vi "read_Rx_pulses_tdms_to data.vi"(8 "error in (no error)":errorcluster, 10 "num of pulses to read":i64=-1, 11 "pulse_gen_and_detect_p2p in":refnum<class "pulse_gen_and_detect_p2p.lvclass">) -> (0 "error out":errorcluster, 2 "PDWout":T1(array[cluster]), 3 "pulse_gen_and_detect_p2p out":refnum<class "pulse_gen_and_detect_p2p.lvclass">)   [LabVIEW 2021, in "pulse_gen_and_detect_p2p.lvclass"]
uses:
  pulse_gen_and_detect_p2p.lvclass
  fpga/vis/pulse detector/PDW interpoter params.ctl
  pulse_gen_and_detect_p2p.lvclass/pulse_gen_and_detect_p2p.ctl
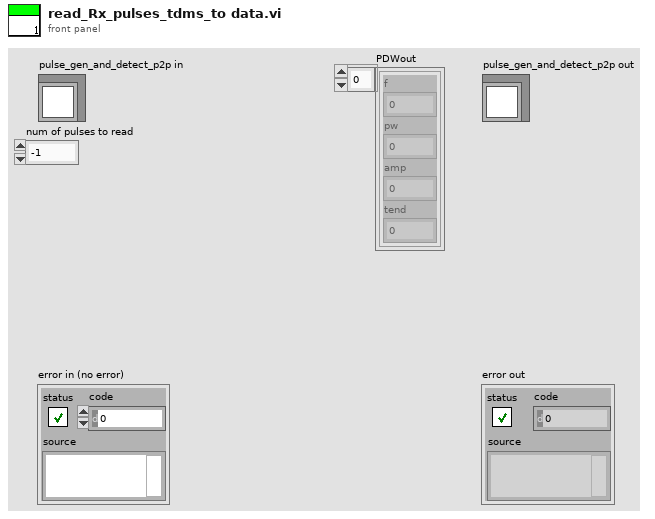
[diagram p1: front panel]
types:
  T1 = cluster{"f":dbl, "pw":dbl, "amp":dbl, "tend":dbl}[]
  T2 = typedef "PDW interpoter params.ctl" = cluster{"Fs (Hz)":dbl, "fft size ":u32, "F base (Hz)":dbl, "min AMP (dB)":dbl, "PW low bar (fft cycle)":dbl, "Pw high bar (fft cycle)":dbl, "lo likege removal (fft bin)":i32, "max gap (fft cycle)":dbl}
  T3 = enum16{"open", "open or create", "create or replace", "create", "open (read-only)"}
  T4 = cluster{"min PW (fft cycels)":u16, "max PW (fft cycels)":u16, "max gap (fft cycels)":u8, "detection bar (liniar amp)":fxp<+,64,63>, "peak detect":bool}
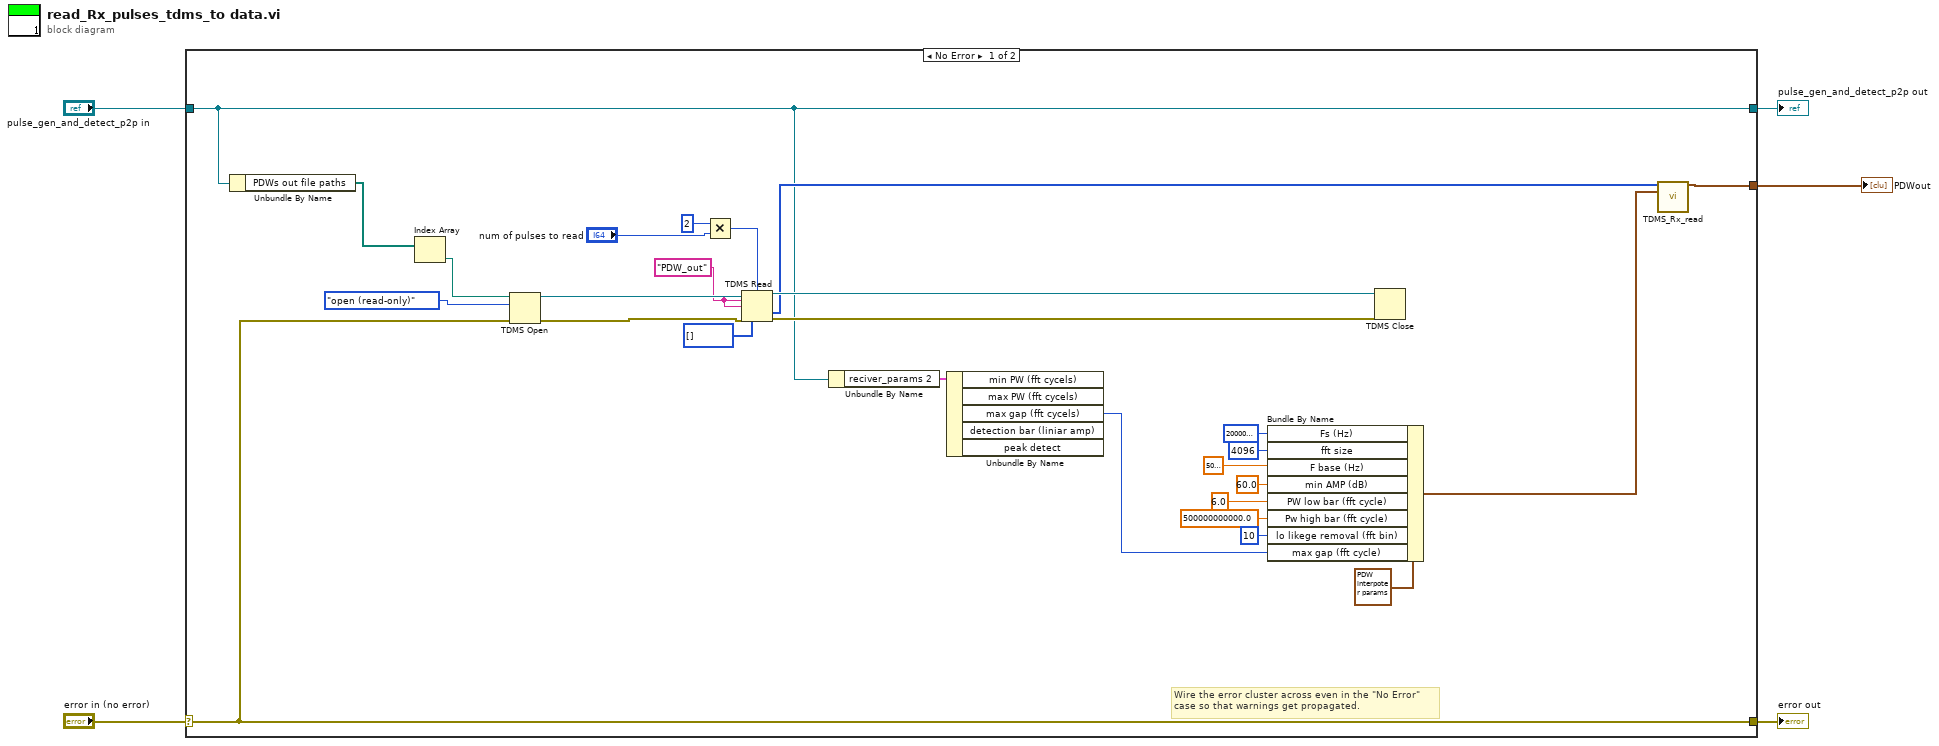
[diagram p0: block diagram]
diagram:
  n1 = case shown="No Error" "error in (no error)" {
    selector: "error in (no error)" -> [w29 w34]
    tunnel: [w29 w34] -> w4
    tunnel: [w9 w33] -> w2
    tunnel: "pulse_gen_and_detect_p2p in" -> [w9 w33]
    tunnel: [w18 _] -> w1
    frame No Error {
      w24 = "PDW_out" ("group name in")
      # "Wire the error cluster across even in the \"No Error\"\ncase so that warnings get propagated."
      n2 = Unbundle By Name(w9) -> ("PDWs out file paths"=w27:path[])
      n3 = Index Array(array=w27) -> (element=w26:path)  [unwired: 1 in]
      n4 = TDMS Open(8:w29, 10:T3."open (read-only)" ("operation (0:open)"), 11:w26) -> (0:w28:errorcluster, 3:w32:refnum<k34>)  [unwired: 4 in]
      n5 = Multiply(x=i64 2, y="num of pulses to read") -> (x*y=w20:i64)
      n6 = TDMS Read(0:w32, 2:w20, 5:w24, 7:w24, 11:w28, 12:u64[] []) -> (4:w31:refnum<k34>, 10:w19:u64[], 15:w23:errorcluster)  [unwired: 2 in, 3 out]
      n7 = Unbundle By Name(w9) -> ("reciver_params 2"=w17:T4)
      n8 = Unbundle By Name(w17) -> ("max gap (fft cycels)"=w14:u8)  [unwired: 4 out]
      n9 = Bundle By Name(cluster=T2 {"Fs (Hz)"=200000000.0, "fft size "=4096, "F base (Hz)"=2000000000.0, "min AMP (dB)"=0.0, "PW low bar (fft cycle)"=0.0, "Pw high bar (fft cycle)"=7000.0, "lo likege removal (fft bin)"=-1, "max gap (fft cycle)"=0.0} ("PDW interpoter params"), "Fs (Hz)"=u32 200000000, "fft size"=u32 4096, "F base (Hz)"=5000000000.0, "min AMP (dB)"=60.0, "PW low bar (fft cycle)"=6.0, "Pw high bar (fft cycle)"=500000000000.0, "lo likege removal (fft bin)"=10, "max gap (fft cycle)"=w14) -> (w8:T2)
      n10 = TDMS Close(8:w23, 11:w31) -> ()  [unwired: 2 out]
      n11 = call "TDMS_Rx_read.vi"("Array in"=w19, "PDW interpoter params"=w8) -> ("Array"=w18:T1)  [unwired: 11 in, 2 out]
    }
    frame Error {
    }
  }
  "error out" <- w4
  "pulse_gen_and_detect_p2p out" <- w2
  "PDWout" <- w1
